vi "Set Scales.vi"(8 "error in (no error)":errorcluster, 10 "Values in":sgl[](array[numeric]), 11 "Barcode Detector in":refnum<class "Barcode Detector.lvclass">) -> (0 "error out":errorcluster, 3 "Barcode Detector":refnum<class "Barcode Detector.lvclass">)   [LabVIEW 2020, in "feature_detection.lvlib" / "Barcode Detector.lvclass"]
uses:
  Barcode Detector.lvclass
  Barcode Detector.lvclass/Barcode Detector.ctl
  <vilib>/Utility/error.llb/Error Cluster From Error Code.vi
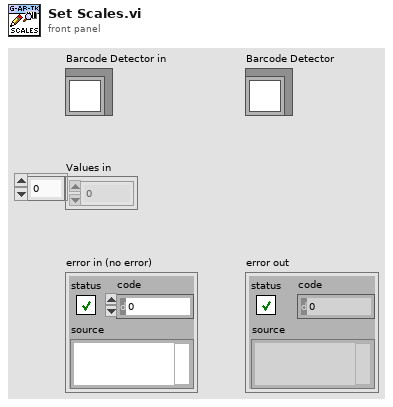
[diagram p1: front panel]
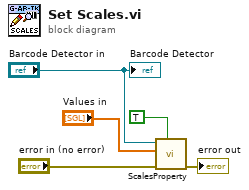
[diagram p0: block diagram]
diagram:
  n1 = call "ScalesProperty.vi"("Write?"=TRUE, "error in (no error)"="error in (no error)", "Values in"="Values in", "Barcode Detector in"="Barcode Detector in") -> ("error out"=→"error out":errorcluster)  [unwired: 6 in, 1 out]
  "Barcode Detector" <- "Barcode Detector in"
